vi "WaitForEdge_MultipleChannels.vi"(4 "Timeout (msec)":i32, 5 "Edge":enum16{"Rising", "Falling", "Both"}(ring), 6 "Bounce time (msec)":i32, 7 "Channels":i32[](array[numeric]), 8 "error in":errorcluster) -> (0 "error out":errorcluster, 3 "Channel out":i32)   [LabVIEW 2014]
doc: "Waits for a specified edge on any of the input channels. Channel out is the number of the first detected edge, or -1 if the wait times out.\n\nAll channels must be configured as an input before calling this VI."
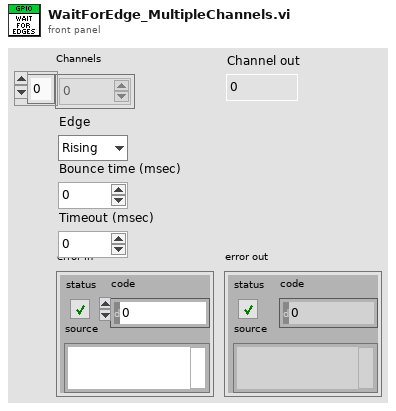
[diagram p1: front panel]
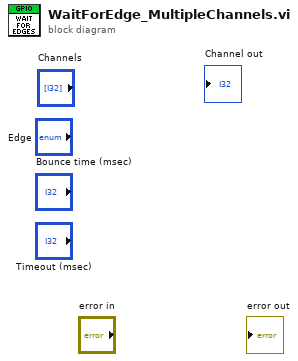
[diagram p0: block diagram]
diagram:
